vi "S2C_BldExitSubScr.vi"(8 "Error In":errorcluster) -> (0 "Error Out":errorcluster)   [LabVIEW 2015]
doc: "Deletes the selected items from the script table."
uses:
  Globals/S2C_Globals.vi
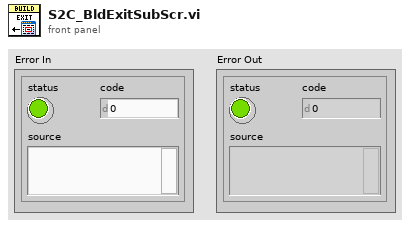
[diagram p1: front panel]
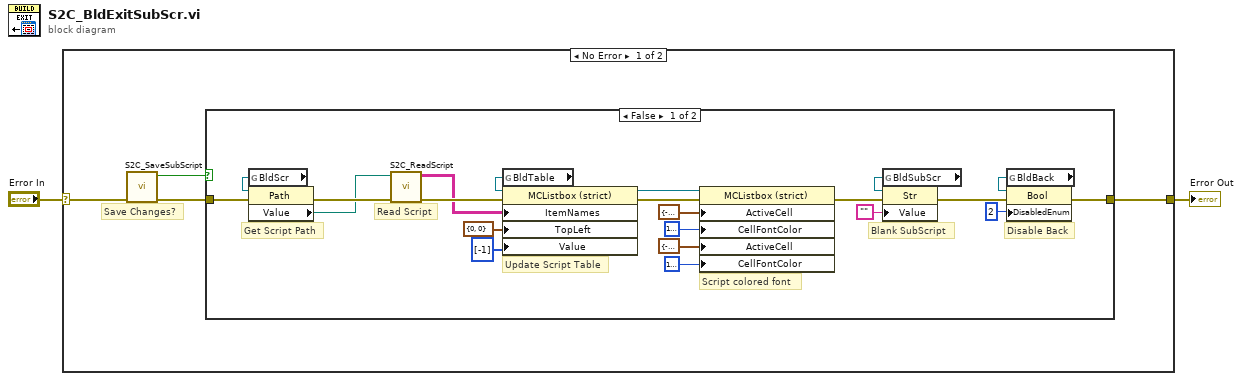
[diagram p0: block diagram]
diagram:
  n1 = case shown="No Error" "Error In" {
    selector: "Error In" -> [w5 w30]
    tunnel: [w6 w30] -> w1
    frame No Error {
      # "Save Changes?"
      n2 = call "S2C_SaveSubScript.vi"("Error In"=w5) -> ("Error Out"=w4:errorcluster, "Cancel?"=w3:bool)  [unwired: 9 in]
      n3 = case shown="False" w3 {
        tunnel: [w28 w29] -> w6
        tunnel: w4 -> [w7 w29]
        frame False {
          # "Read Script"
          # "Script colored font"
          # "Get Script Path"
          # "Update Script Table"
          # "Disable Back"
          # "Blank SubScript"
          n4 = global read "S2C_Globals.vi" "BldScr"() -> (w20:refnum<vi>)
          n5 = property class="Path"(reference=w20, error in=w7) -> (error out=w11:errorcluster, "Value"=w10:path)  [unwired: 1 out]
          n6 = call "S2C_ReadScript.vi"("Error In"=w11, "FilePath"=w10) -> ("Error Out"=w9:errorcluster, "Data"=w8:string[][])  [unwired: 8 in]
          n7 = global read "S2C_Globals.vi" "BldTable"() -> (w27:refnum<vi>)
          n8 = property class="MCListbox (strict)"(reference=w27, error in=w9, "ItemNames"=w8, "TopLeft"=cluster{"Row":u32, "Column":u32} {"Row"=0, "Column"=0} ("Top Left Visible Cell"), "Value"=i32[] [-1]) -> (reference out=w13:refnum<vi>, error out=w14:errorcluster)
          n9 = property class="MCListbox (strict)"(reference=w13, error in=w14, "ActiveCell"=cluster{"Row":i32, "Column":i32} {"Row"=-2, "Column"=-2} ("Active Cell:Active Cell"), "CellFontColor"=u32 16777222, "ActiveCell"=cluster{"Row":i32, "Column":i32} {"Row"=-1, "Column"=-2} ("Active Cell:Active Cell"), "CellFontColor"=u32 16777226) -> (error out=w12:errorcluster)  [unwired: 1 out]
          n10 = global read "S2C_Globals.vi" "BldSubScr"() -> (w24:refnum<vi>)
          n11 = property class="Str"(reference=w24, error in=w12, "Value"="") -> (error out=w22:errorcluster)  [unwired: 1 out]
          n12 = global read "S2C_Globals.vi" "BldBack"() -> (w23:refnum<vi>)
          n13 = property class="Bool"(reference=w23, error in=w22, "DisabledEnum"=u8 2) -> (error out=w28:errorcluster)  [unwired: 1 out]
        }
        frame True {
        }
      }
    }
    frame Error {
    }
  }
  "Error Out" <- w1
